vi "55 Channels.vi"() -> ()   [LabVIEW 2019]
uses:
  <extravilib>/ChannelInstances/Tag-i32.lvlib
  _Subs/OpenDiagram/Open_XControl.xctl
panel:
  in  "OpenDiag":refnum<vi>(xcontrol)
  out "Reader i":i32
  out "Writer i":i32
  out "Reader":i32(graph)
  in  "Stop":bool
  out "Writer":i32(graph)
  # "05 Channels\nThis code shows data shared across two parallel loops\n\nInstructions:\n1. Hit the Run arrow and see two loops run at the same time, sharing data"
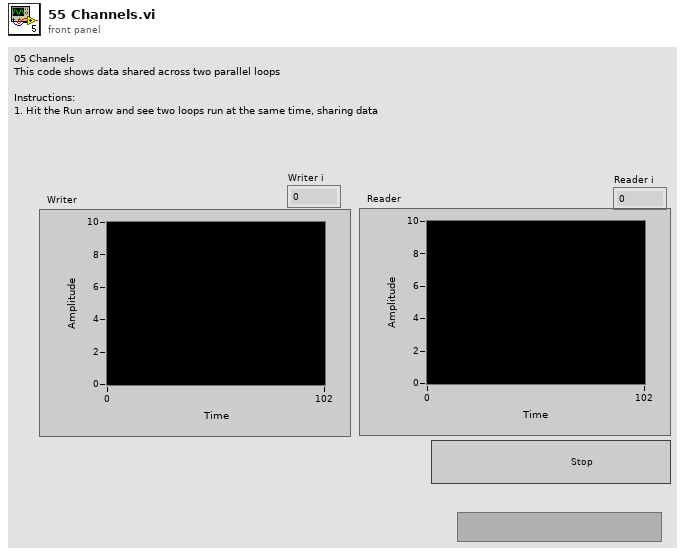
[diagram p1: front panel]
types:
  T1 = typedef "Tag-i32.lvlib/))Channel.ctl" = refnum<queue>
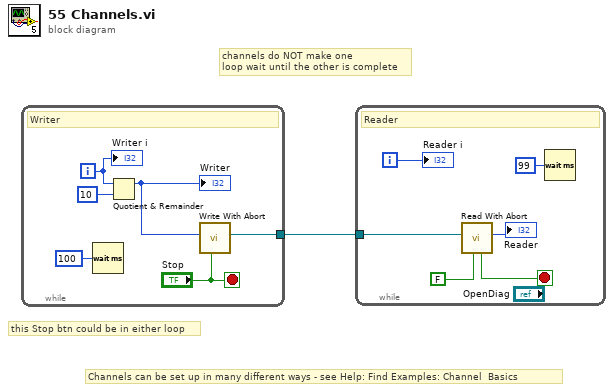
[diagram p0: block diagram]
diagram:
  # "channels do NOT make one \nloop wait until the other is complete"
  # "Channels can be set up in many different ways - see Help: Find Examples: Channel  Basics"
  # "this Stop btn could be in either loop"
  n1 = while {
    tunnel: [w3] -> w1
    i -> [w6]
    stop <- "Stop" stop-if-true
    # "Writer"
    n2 = Wait (ms)(milliseconds to wait=u32 100) -> ()  [unwired: 1 out]
    n3 = Quotient & Remainder(x=w6, y=10) -> (x-y*floor(x/y)=w5:i32)  [unwired: 1 out]
    "Writer" <- w5
    n4 = call <extravilib>:"Write With Abort.vi"("abort"="Stop", "element"=w5) -> ("channel"=w3:T1)  [unwired: 7 in, 2 out]
    "Writer i" <- w6
  }
  n5 = while {
    tunnel: w1 -> [w11]
    i -> [w9]
    stop <- w13 stop-if-true
    # "Reader"
    n6 = call <extravilib>:"Read With Abort.vi"("abort"=FALSE, "channel"=w11) -> ("element"=→"Reader":i32, "aborted?"=w13:bool)  [unwired: 7 in, 1 out]
    n7 = Wait (ms)(milliseconds to wait=u32 99) -> ()  [unwired: 1 out]
    "Reader i" <- w9
  }
